vi "SplitHTTPHeaders.vi"(8 "error in (no error)":errorcluster, 11 "HTTP Header String":string) -> (0 "error out":errorcluster, 2 "Headers Array":string[][](array[string]), 3 "HTTP Request":string)   [LabVIEW 2012, in "WebSockets.lvlib"]
doc: "Returns the remaining HTTP headers received from the client."
uses:
  WebSockets.lvlib
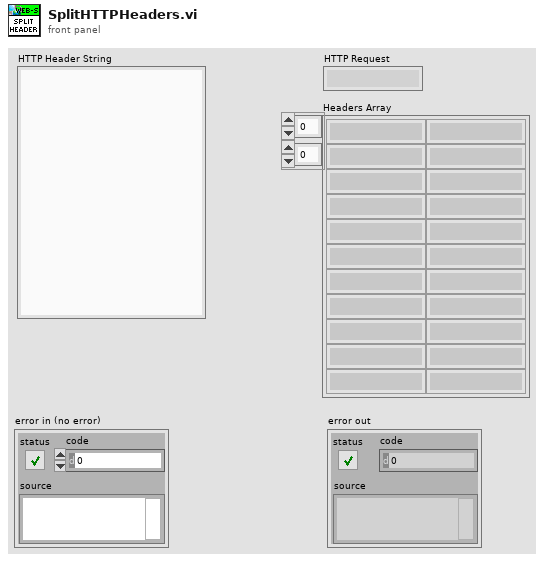
[diagram p1: front panel]
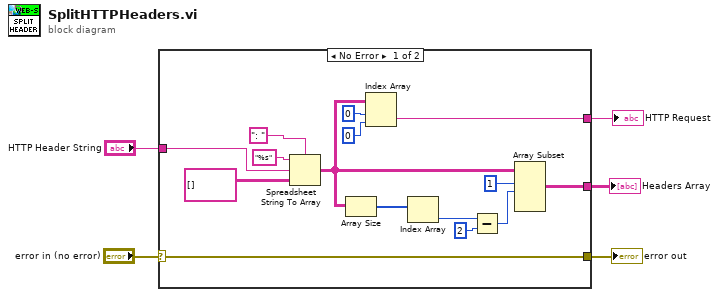
[diagram p0: block diagram]
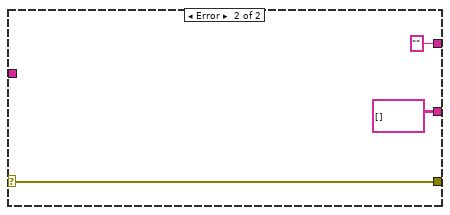
[diagram p2: hidden frame]
diagram:
  n1 = case shown="No Error" "error in (no error)" {
    selector: "error in (no error)" -> [w6 w23]
    tunnel: [w20 string[][] []] -> w5
    tunnel: [w19 ""] -> w4
    tunnel: "HTTP Header String" -> [w8 _]
    tunnel: [w6 w23] -> w1
    frame No Error {
      n2 = Spreadsheet String To Array(delimiter (Tab)=": ", format string="%s", spreadsheet string=w8, array type (2D Dbl)=string[][] []) -> (array=w14:string[][])
      n3 = Array Size(array=w14) -> (size(s)=w15:i32[])
      n4 = Index Array(array=w14, index (row)=0, index (col)=0 ("disabled index (col)")) -> (element=w19:string)
      n5 = Index Array(array=w15) -> (element=w16:i32)  [unwired: 1 in]
      n6 = Subtract(x=w16, y=2) -> (x-y=w17:i32)
      n7 = Array Subset(array=w14, index (row)=1 ("index"), length (row)=w17) -> (w20:string[][])  [unwired: 2 in]
    }
    frame Error {
    }
  }
  "Headers Array" <- w5
  "HTTP Request" <- w4
  "error out" <- w1
